vi "addData.vi"(0 "U8ArrayBuilderManualIndexing in":refnum<class "U8ArrayBuilderManualIndexing.lvclass">, 5 "Data":u8[](array[numeric]), 7 "Index":i32, 9 "OverrideSwapBytes":bool, 11 "error in (no error)":errorcluster) -> (4 "U8ArrayBuilderManualIndexing out":refnum<class "U8ArrayBuilderManualIndexing.lvclass">, 6 "Index out":i32, 15 "error out":errorcluster)   [LabVIEW 2016, in "RTUtilities.lvlib" / "U8ArrayBuilderManualIndexing.lvclass"]
uses:
  U8ArrayBuilderManualIndexing.lvclass
  U8ArrayBuilderManualIndexing.lvclass/U8ArrayBuilderManualIndexing.ctl
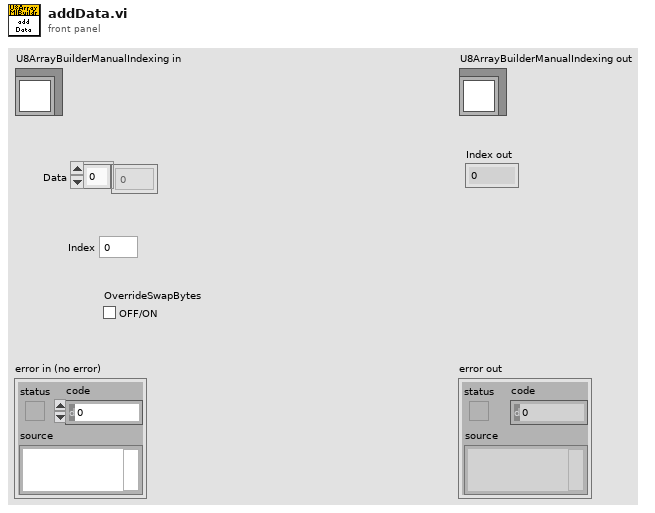
[diagram p1: front panel]
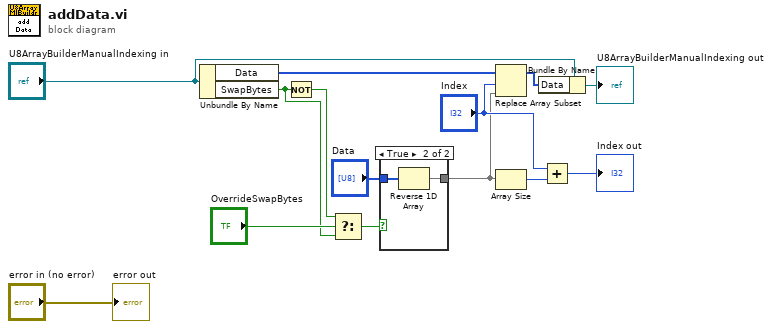
[diagram p0: block diagram]
diagram:
  n1 = Unbundle By Name("U8ArrayBuilderManualIndexing in") -> ("Data"=w11:u8[], "SwapBytes"=w6:bool)
  n2 = Not(x=w6) -> (.not. x?=w7:bool)
  n3 = Select(t=w7, s="OverrideSwapBytes", f=w6) -> (s? t:f=w5:bool)
  n4 = case shown="True" w5 {
    tunnel: "Data" -> [w15 w17]
    tunnel: [w15 w16] -> w2
    frame False {
    }
    frame True {
      n5 = Reverse 1D Array(array=w17) -> (reversed array=w16:u8[])
    }
  }
  n6 = Replace Array Subset(array=w11, new element=w2, index="Index") -> (w10:u8[])
  n7 = Array Size(array=w2) -> (size(s)=w3:i32)
  n8 = Bundle By Name(cluster="U8ArrayBuilderManualIndexing in", "Data"=w10) -> (→"U8ArrayBuilderManualIndexing out":refnum<class "U8ArrayBuilderManualIndexing.lvclass">)
  n9 = Add(x="Index", y=w3) -> (x+y=→"Index out":i32)
  "error out" <- "error in (no error)"
